vi "VisualiseDiscData.vi"(11 "DiscData":i64[](array[numeric])) -> (3 "result string":string)   [LabVIEW 2023, in "2024_9.lvclass"]
uses:
  2024_9.lvclass
  2024_9.lvclass/2024_9.ctl
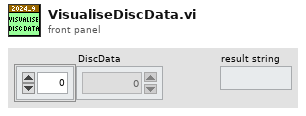
[diagram p1: front panel]
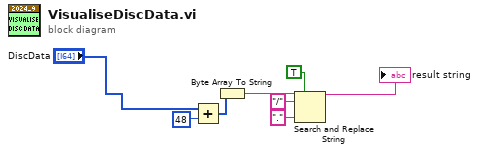
[diagram p0: block diagram]
diagram:
  n1 = Add(x="DiscData", y=48) -> (x+y=w3:i64[])
  n2 = Byte Array To String(unsigned byte array=w3) -> (string=w4:string)
  n3 = Search and Replace String(replace all?=TRUE ("replace all? (F)"), input string=w4, search string="/", replace string="." ("replace string (\"\")")) -> (result string=→"result string":string)  [unwired: 4 in, 3 out]
